vi "顺序结构（匹配数字计时）.vi"() -> ()   [LabVIEW 2017]
panel:
  in  "预设整数":dbl
  out "循环次数":i32
  out "用时（ms）":u32
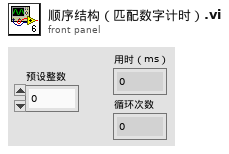
[diagram p1: front panel]
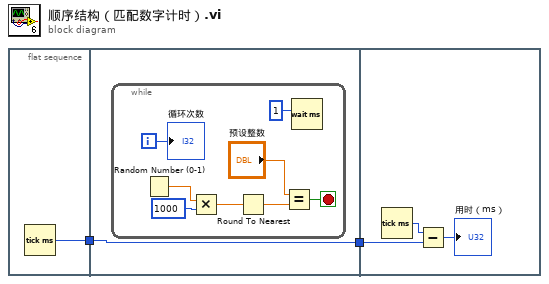
[diagram p0: block diagram]
diagram:
  n1 = flat-sequence {
    tunnel: [w3] -> w2
    tunnel: w2 -> [w4]
    tunnel: [w4] -> w1
    tunnel: w1 -> [w14]
    frame #0 {
      n2 = Tick Count (ms)() -> (millisecond timer value=w3:u32)
    }
    frame #1 {
      n3 = while {
        i -> [w12]
        stop <- w8 stop-if-true
        n4 = Random Number (0-1)() -> (number: 0 to 1=w11:dbl)
        n5 = Multiply(x=w11, y=1000) -> (x*y=w9:dbl)
        n6 = Round To Nearest(number=w9) -> (nearest integer value=w6:dbl)
        n7 = Equal?(x="预设整数", y=w6) -> (x = y?=w8:bool)
        n8 = Wait (ms)(milliseconds to wait=u32 1 ("等待时间（毫秒）")) -> ()  [unwired: 1 out]
        "循环次数" <- w12
      }
    }
    frame #2 {
      n9 = Tick Count (ms)() -> (millisecond timer value=w15:u32)
      n10 = Subtract(x=w15, y=w14) -> (x-y=→"用时（ms）":u32)
    }
  }
